vi "Add Process.vi"(8 "error in (no error)":errorcluster, 10 "Debug Process":refnum<class "Debug Process.lvclass">, 11 "Main In":refnum<class "Main.lvclass">) -> (0 "error out":errorcluster, 3 "Main Out":refnum<class "Main.lvclass">)   [LabVIEW 2020, in "Main.lvclass"]
uses:
  Main.lvclass
  Process/Debug Process.lvclass
  Main.lvclass/Main.ctl
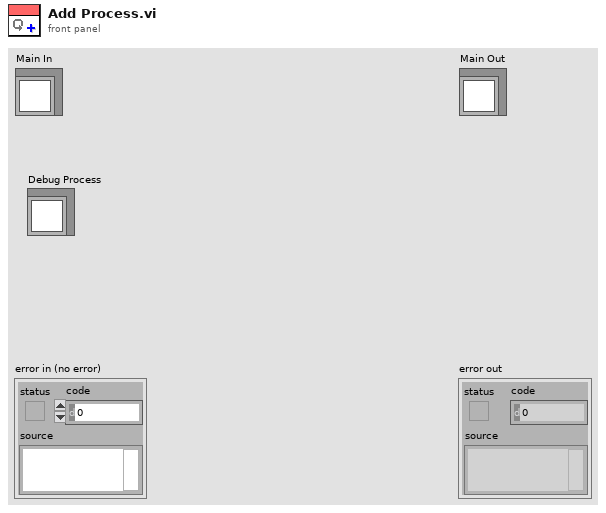
[diagram p1: front panel]
types:
  T1 = map{string, refnum<class "Debug Process.lvclass">}
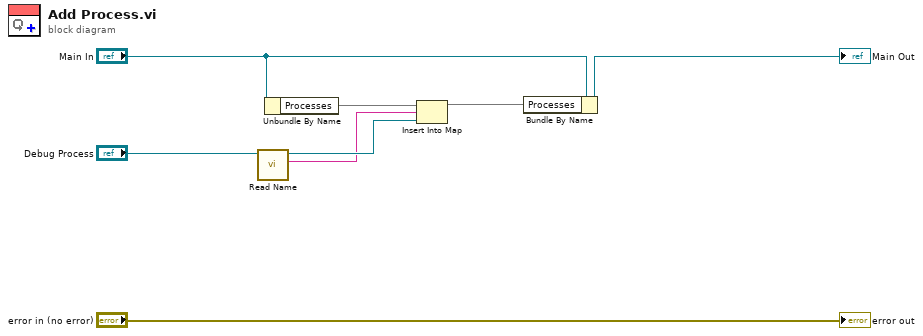
[diagram p0: block diagram]
diagram:
  n1 = call "Read Name.vi"("Process In"="Debug Process") -> ("Name"=w1:string, "Process Out"=w2:refnum<class "Debug Process.lvclass">)  [unwired: 8 in, 1 out]
  n2 = Unbundle By Name("Main In") -> ("Processes"=w4:T1)
  n3 = Insert Into Map(map in=w4, key=w1, value=w2) -> (map out=w3:T1)  [unwired: 2 out]
  n4 = Bundle By Name(cluster="Main In", "Processes"=w3) -> (→"Main Out":refnum<class "Main.lvclass">)
  "error out" <- "error in (no error)"
